vi "Test Left Menu Disabled at Card Inserted.vi"(8 "error in (no error)":errorcluster, 11 "Test Case In":refnum<class "View Model Test.lvclass">) -> (0 "error out":errorcluster, 3 "Test Case Out":refnum<class "View Model Test.lvclass">)   [LabVIEW 2020, in "View Model Test.lvclass"]
uses:
  View Model Test.lvclass
  View Model Test.lvclass/View Model Test.ctl
  01074fa8-ee8a-411d-bc8b-fc92c4f90959.vi
  ATM View Model/ATM View Model.lvclass
  ATM View Model/Controls.ctl
  ATM Controller/State.ctl
  ATM Controller/ATM Controller.lvclass
panel:
  out "Test Control":bool
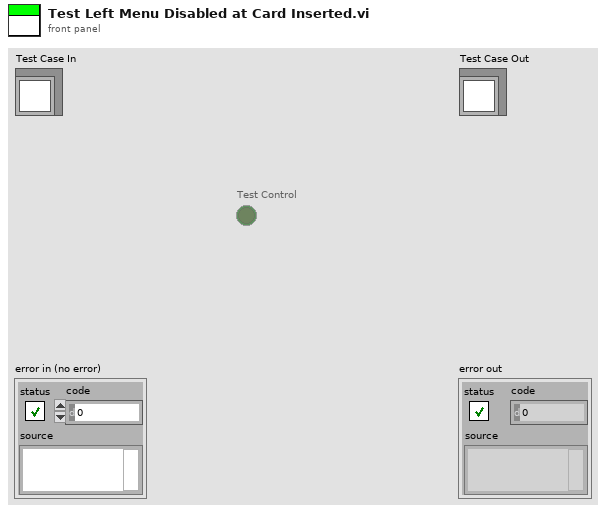
[diagram p1: front panel]
types:
  T1 = enum8{"Enabled", "Disabled", "Disabled and Grayed Out"}
  T2 = typedef "ATM Controller.lvclass/State.ctl" = enum16{"Start", "Card Inserted", "Verification Failed", "Verification Succeeded", "Depositing", "Depositing Completed", "Withdrawing", "Withdraw Completed", "Withdraw Failed", "Balance Inquiry", "Terminate"}
  T3 = typedef "ATM View Model.lvclass/Controls.ctl" = enum16{"User Input", "Enter", "Left Menu", "Right Menu", "Left Button", "Right Button", "Card Simulator"}
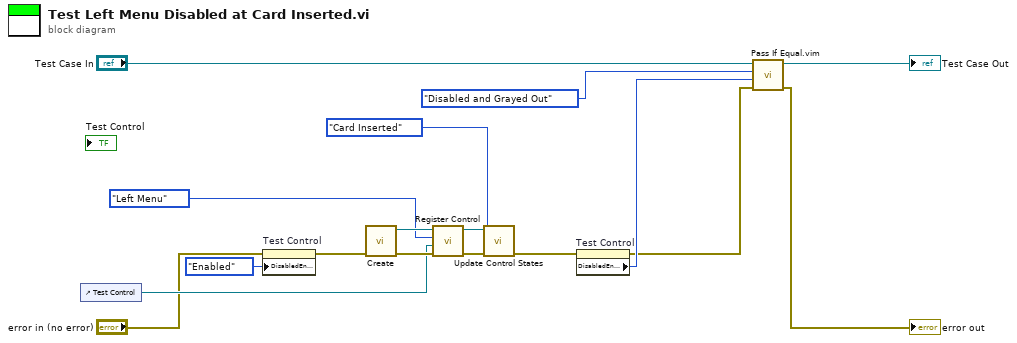
[diagram p0: block diagram]
diagram:
  n1 = control-ref of="Test Control"() -> (w9:refnum<vi>)
  n2 = property on="Test Control" class="Bool (strict)"(error in="error in (no error)", "DisabledEnum"=T1."Enabled" ("Disabled")) -> (error out=w2:errorcluster)  [unwired: 1 in, 1 out]
  n3 = call "Create.vi"("error in (no error)"=w2) -> ("error out"=w12:errorcluster, "ATM View Model out"=w13:refnum<class "ATM View Model.lvclass">)  [unwired: 9 in]
  n4 = call "Register Control.vi"("error in (no error)"=w12, "Control ref"=w9, "Control"=Controls."Left Menu" ("Controls"), "ATM View Model in"=w13) -> ("error out"=w10:errorcluster, "ATM View Model out"=w11:refnum<class "ATM View Model.lvclass">)  [unwired: 6 in]
  n5 = call "Update Control States.vi"("error in (no error)"=w10, "ATM State"=State."Card Inserted", "ATM View Model In"=w11) -> ("error out"=w7:errorcluster)  [unwired: 7 in, 1 out]
  n6 = property on="Test Control" class="Bool (strict)"(error in=w7) -> (error out=w5:errorcluster, "DisabledEnum"=w6:T1)  [unwired: 1 in, 1 out]
  n7 = call "Pass If Equal.vim"("error in (no error)"=w5, "Actual"=w6, "Expected"=T1."Disabled and Grayed Out" ("Enable State"), "LUnit Test Case In"="Test Case In") -> ("error out"=→"error out":errorcluster, "LUnit Test Case Out"=→"Test Case Out":refnum<class "View Model Test.lvclass">)  [unwired: 6 in]
